vi "Create Client.vi"(8 "error in":errorcluster, 10 "certificatePath":string, 11 "address":string) -> (0 "error out":errorcluster, 3 "ClientID out":T1)   [LabVIEW 2019, in "grpc-lvsupport.lvlib"]
uses:
  grpc-lvsupport.lvlib
  grpcId.ctl
  <vilib>/Utility/error.llb/Error Cluster From Error Code.vi
  <resource>/libgrpc_labview.dll
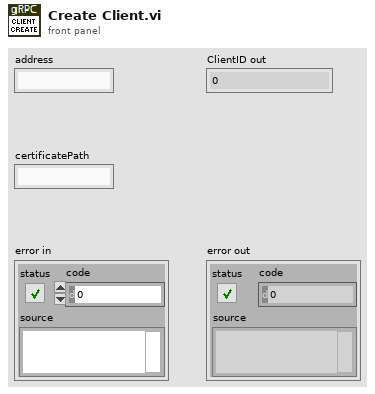
[diagram p1: front panel]
types:
  T1 = typedef "grpc-lvsupport.lvlib/grpcId.ctl" = u64
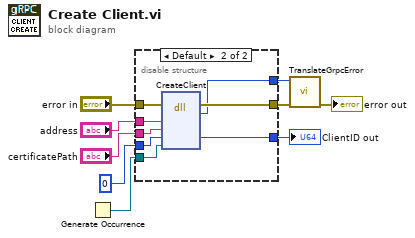
[diagram p0: block diagram]
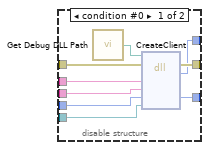
[diagram p2: hidden frame]
diagram:
  n1 = Generate Occurrence() -> (w1:refnum<k4>)
  n2 = disable-structure shown="Default" {
    disable-tunnel: [w18 w26] -> w2
    disable-tunnel: [w16 w25] -> w9
    disable-tunnel: "address" -> [w15 w24]
    disable-tunnel: "certificatePath" -> [w14 w23]
    disable-tunnel: [w13 w22] -> w5
    disable-tunnel: "error in" -> [w12 w21]
    disable-tunnel: u64 0 ("clientId") -> [w11 w20]
    disable-tunnel: w1 -> [w10 w19]
    frame condition #0 {
      n3 = call "Get Debug DLL Path.vi"() -> ("DLL Path"=w17:path)
      n4 = dll-call lib="?" fn="CreateClient"(path in=w17, error in=w12, "address"=w15, "certificatePath"=w14, "clientId"=w11, "InitCallbackOccurrence"=w10) -> (error out=w18:errorcluster, "return type"=w13:i32, "clientId"=w16:u64)  [unwired: 4 in, 1 out]
    }
    frame condition #1 (active) {
      n5 = dll-call lib="C:/Program Files (x86)/National Instruments/LabVIEW 2024/resource/libgrpc_labview.*" fn="CreateClient"(error in=w21, "address"=w24, "certificatePath"=w23, "clientId"=w20, "InitCallbackOccurrence"=w19) -> (error out=w26:errorcluster, "return type"=w22:i32, "clientId"=w25:u64)  [unwired: 5 in, 1 out]
    }
  }
  "ClientID out" <- w9
  n6 = call "TranslateGrpcError.vi"("error in"=w2, "Error Code"=w5) -> ("error out"=→"error out":errorcluster)  [unwired: 9 in]
